vi "DVR Creator.vi"(0 "Numeric Input":dbl=5.0, 5 "Increment":bool, 7 "Stop":bool, 11 "Error In":errorcluster) -> (15 "Error Out":errorcluster)   [LabVIEW 2023]
doc: "The VI creates a DVR for the numeric value and stores it in a functional global, clicking increment will increment the value by one on each click and stops the VI on clicking stop button."
uses:
  Controls/Operation.ctl
panel:
  # "Instructipons:\n1. Run the VI.\n2. Run the DVR Reader.vi to get the values.\n3. Click increment to increase the value of the DVR by one.\n4. Press stop button or panel close to stop the VI."
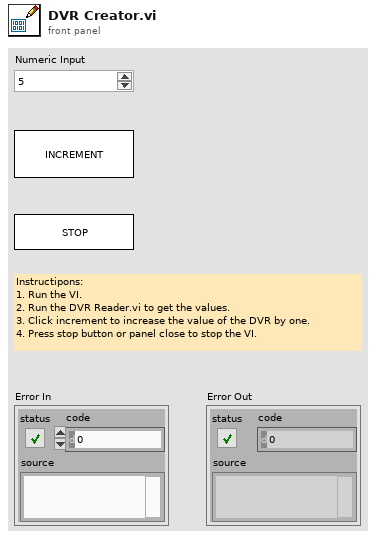
[diagram p1: front panel]
types:
  T1 = enum8{"Enabled", "Disabled", "Disabled and Grayed Out"}
  T2 = typedef "Operation.ctl" = enum16{"Write Ref", "Read Ref"}
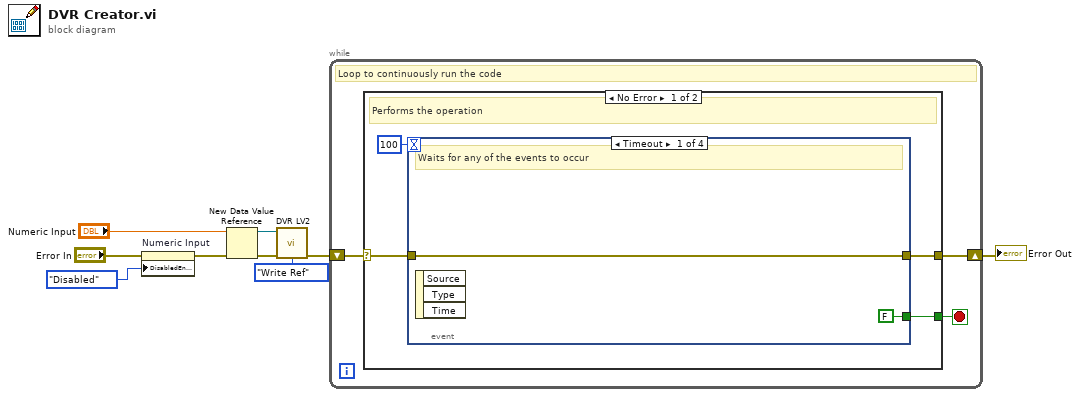
[diagram p0: block diagram]
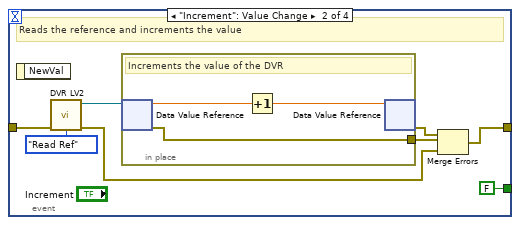
[diagram p2: hidden frame]
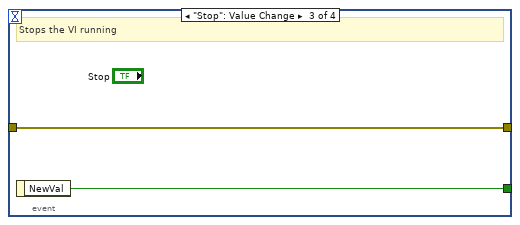
[diagram p3: hidden frame]
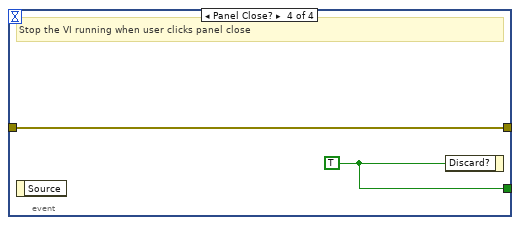
[diagram p4: hidden frame]
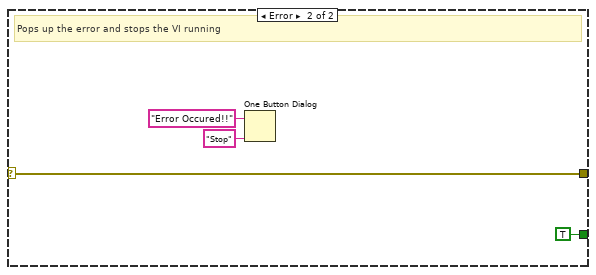
[diagram p5: hidden frame]
diagram:
  n1 = property on="Numeric Input" class="DigNum (strict)"(error in="Error In", "DisabledEnum"=T1."Disabled" ("Disabled")) -> (error out=w2:errorcluster)  [unwired: 1 in, 1 out]
  n2 = New Data Value Reference(data value="Numeric Input", error in=w2) -> (data value reference=w4:refnum<data-value>, error out=w7:errorcluster)
  n3 = call "DVR LV2.vi"("Data Value Refnum In"=w4, "Error In"=w7, "Operation"=Operation."Write Ref") -> ("Error Out"=w6:errorcluster)  [unwired: 11 in, 1 out]
  n4 = while {
    shift-right: [w12] -> w8
    shift-left: w6 -> [w10]
    stop <- w11 stop-if-true
    # "Loop to continuously run the code"
    n5 = case shown="No Error" w10 {
      selector: w10 -> [w13 w37]
      tunnel: [w16 w37] -> w12
      tunnel: [w14 TRUE ("Discard?")] -> w11
      frame No Error {
        # "Performs the operation"
        n6 = event shown="[0] Timeout" {
          selector: _ -> [_ _ _ _]
          dyn-events: _ -> [_ _ _ _]
          timeout: 100 -> [_ _ _ _]
          tunnel: [w17 w19 w30 w32] -> w16
          tunnel: [FALSE ("Discard?") FALSE ("Discard?") w31 w33] -> w14
          tunnel: w13 -> [w17 w26 w30 w32]
          event Timeout {
            # "Waits for any of the events to occur"
            n7 = event-data() -> ()  [unwired: 1 in, 3 out]
          }
          event "Increment": Value Change {
            # "Reads the reference and increments the value"
            n8 = event-data() -> ()  [unwired: 1 in, 1 out]
            n9 = call "DVR LV2.vi"("Error In"=w26, "Operation"=Operation."Read Ref") -> ("Data Value Refnum Out"=w24:refnum<data-value>, "Error Out"=w21:errorcluster)  [unwired: 12 in]
            n10 = in-place {
              in-place-border: [w27] -> w22
              # "Increments the value of the DVR"
              n11 = in-place-dvr #1(w24) -> (w29:dbl, w27:errorcluster)
              n12 = Increment(x=w29) -> (x+1=w28:dbl)
              n13 = in-place-dvr #1(w28) -> (w20:errorcluster)  [unwired: 1 out]
            }
            n14 = Merge Errors(w20, w22, w21) -> (w19:errorcluster)
          }
          event "Stop": Value Change {
            # "Stops the VI running"
            n15 = event-data() -> ("NewVal"=w31:bool)  [unwired: 1 in]
          }
          event Panel Close? {
            w33 = TRUE ("Discard?")
            # "Stop the VI running when user clicks panel close"
            n16 = event-data() -> ()  [unwired: 1 in, 1 out]
            n17 = event-data("Discard?"=w33) -> ()  [unwired: 1 in, 1 out]
          }
        }
      }
      frame Error {
        # "Pops up the error and stops the VI running"
        n18 = One Button Dialog(message="Error Occured!!", button name ("OK")="Stop") -> ()  [unwired: 1 out]
      }
    }
  }
  "Error Out" <- w8
